vi "Close Hardware Session.vi"(8 "error in":errorcluster, 11 "hardware handles":T1) -> (0 "error out":errorcluster)   [LabVIEW 2020, in "Ballard MIL-STD-1553 Engine.lvlib" / "Custom Device.lvlib"]
uses:
  Custom Device.lvlib
  Hardware Handles.ctl
  <instrlib>/BTICardLib/BTICardLV.lvlib
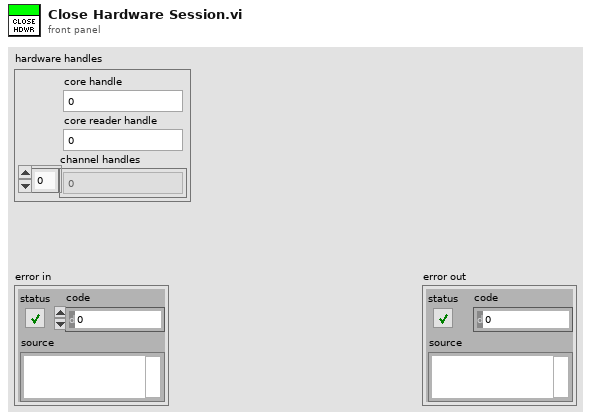
[diagram p1: front panel]
types:
  T1 = typedef "Ballard MIL-STD-1553 Engine.lvlib/Custom Device.lvlib/Hardware Handles.ctl" = cluster{"core handle":u64, "core reader handle":u64, "channel handles":u64[]}
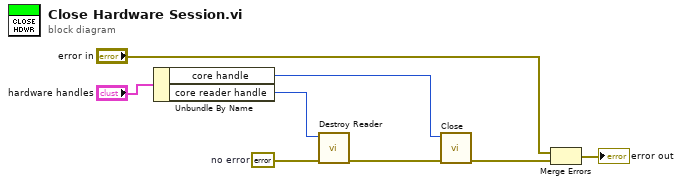
[diagram p0: block diagram]
diagram:
  w7 = errorcluster {"status"=FALSE, "code"=0, "source"=""}  # no error
  n1 = Unbundle By Name("hardware handles") -> ("core handle"=w5:u64, "core reader handle"=w6:u64)
  n2 = call <instrlib>:"Destroy Reader.vi"("error in (no error)"=w7, "reader handle in"=w6) -> ("error out"=w4:errorcluster)  [unwired: 9 in]
  n3 = call <instrlib>:"Close.vi"("error in (no error)"=w4, "core handle in"=w5) -> ("error out"=w3:errorcluster)  [unwired: 8 in, 1 out]
  n4 = Merge Errors("error in", w3) -> (→"error out":errorcluster)
